vi "Write Boolean Text Props.vi"(8 "error in (no error)":errorcluster, 10 "Boolean Text Props":T1, 11 "Control In":refnum<vi>) -> (0 "error out":errorcluster, 3 "Control":refnum<vi>)   [LabVIEW 2020, in "VolatusGUIEditorCore.lvlib"]
uses:
  VolatusGUIEditorCore.lvlib
  Boolean Text Props.ctl
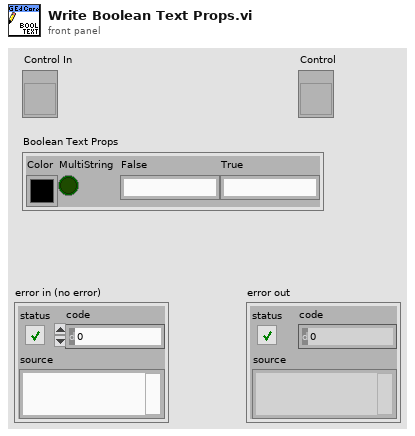
[diagram p1: front panel]
types:
  T1 = typedef "VolatusGUIEditorCore.lvlib/Boolean Text Props.ctl" = cluster{"Color":u32, "MultiString":bool, "False":string, "True":string}
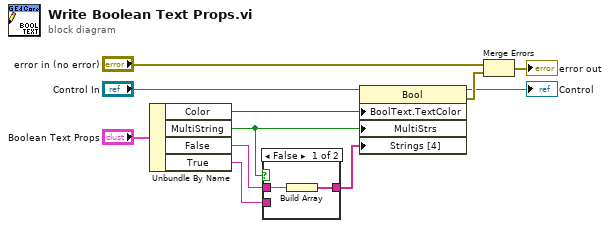
[diagram p0: block diagram]
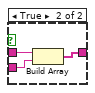
[diagram p2: hidden frame]
diagram:
  n1 = Unbundle By Name("Boolean Text Props") -> ("Color"=w7:u32, "MultiString"=w6:bool, "False"=w10:string, "True"=w9:string)
  n2 = case shown="False" w6 {
    tunnel: w10 -> [w13 w16]
    tunnel: w9 -> [_ w15]
    tunnel: [w12 w14] -> w5
    frame False {
      n3 = Build Array(w13) -> (w12:string[])
    }
    frame True {
      n4 = Build Array(w16, w15) -> (w14:string[])
    }
  }
  n5 = property class="Bool"(reference="Control In", "BoolText.TextColor"=w7, "MultiStrs"=w6, "Strings [4]"=w5) -> (reference out=→"Control":refnum<vi>, error out=w3:errorcluster)  [unwired: 1 in]
  n6 = Merge Errors("error in (no error)", w3) -> (→"error out":errorcluster)
